vi "ConvertVoltToDegree.vi"(10 "Tension":dbl) -> (2 "Température":dbl)   [LabVIEW 2018]
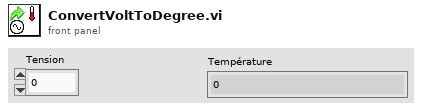
[diagram p1: front panel]
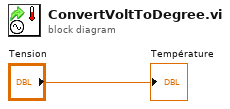
[diagram p0: block diagram]
diagram:
  "Température" <- "Tension"
